vi "main 2.7.22.vi"() -> ()   [LabVIEW 2021]
panel:
  out "Thermistors":cluster{"Filtered x":dbl, "Filtered x":dbl}(graph)
  out "Waveform Chart 3":T1(graph)
  in  "error in (no error)":errorcluster
  out "error out":errorcluster
  out "Waveform Chart 2":waveform(dbl)(graph)
  out "a0 Scalar":dbl
  out "Waveform Chart":dynamicdata(graph)
  in  "stop":bool
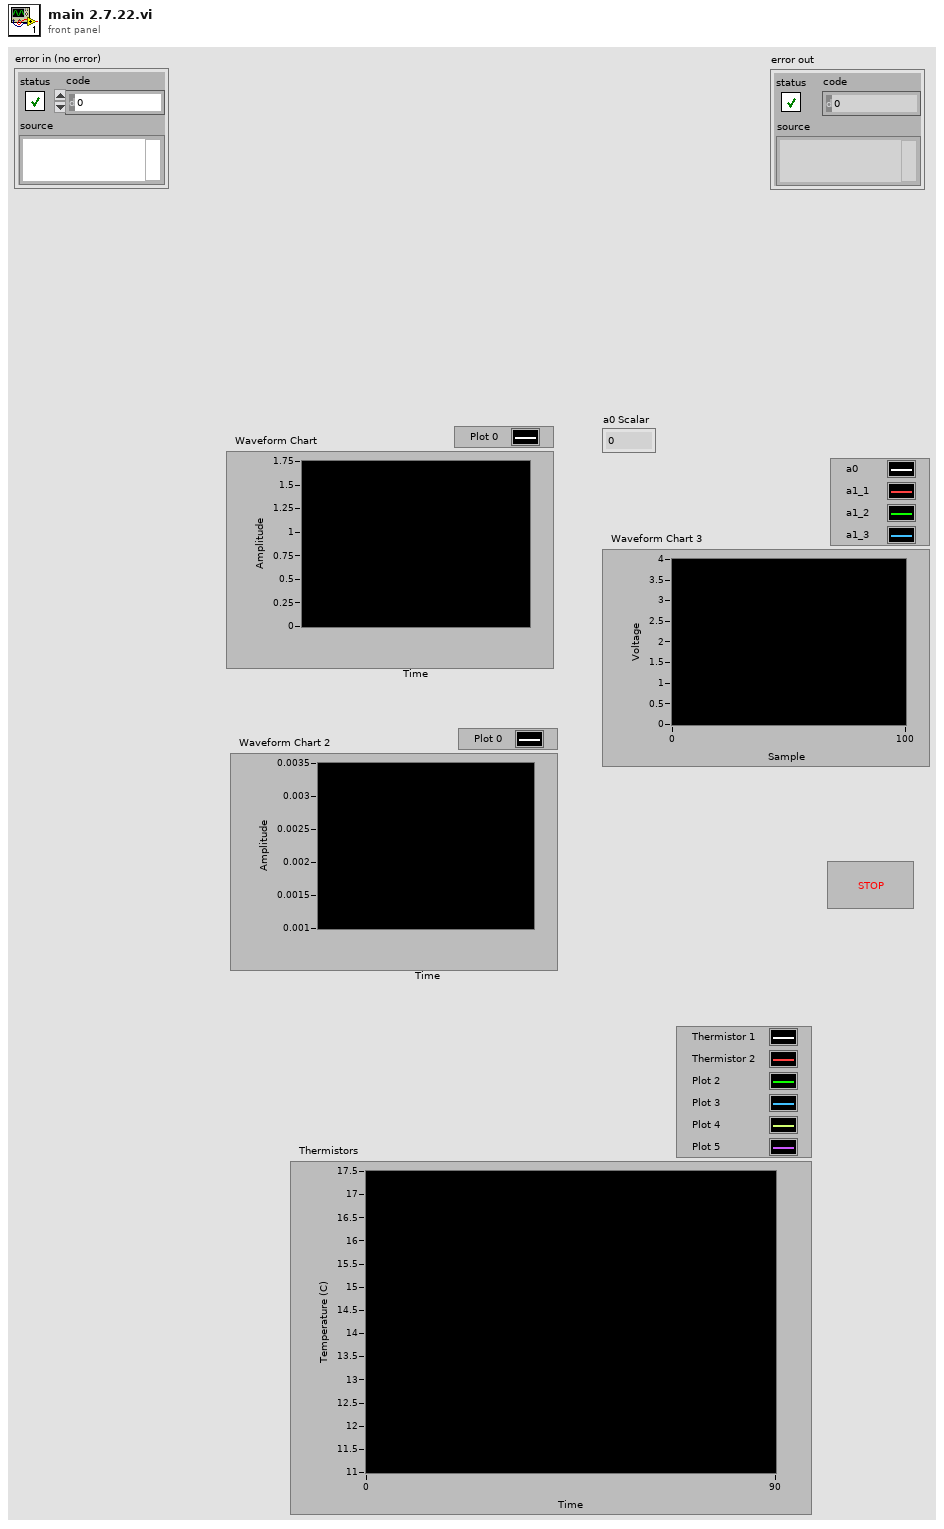
[diagram p1: front panel]
types:
  T1 = cluster{"Data_Array[0]":dbl, "Data_Array[1]":dbl, "Data_Array[2]":dbl, "Data_Array[3]":dbl, "Data_Array[4]":dbl, "Data_Array[5]":dbl, "Data_Array[6]":dbl, "Data_Array[7]":dbl, "Data_Array[8]":dbl}
  T2 = cluster{"Data_Array":dbl[], "Multiplex_Tbl":u32[]}
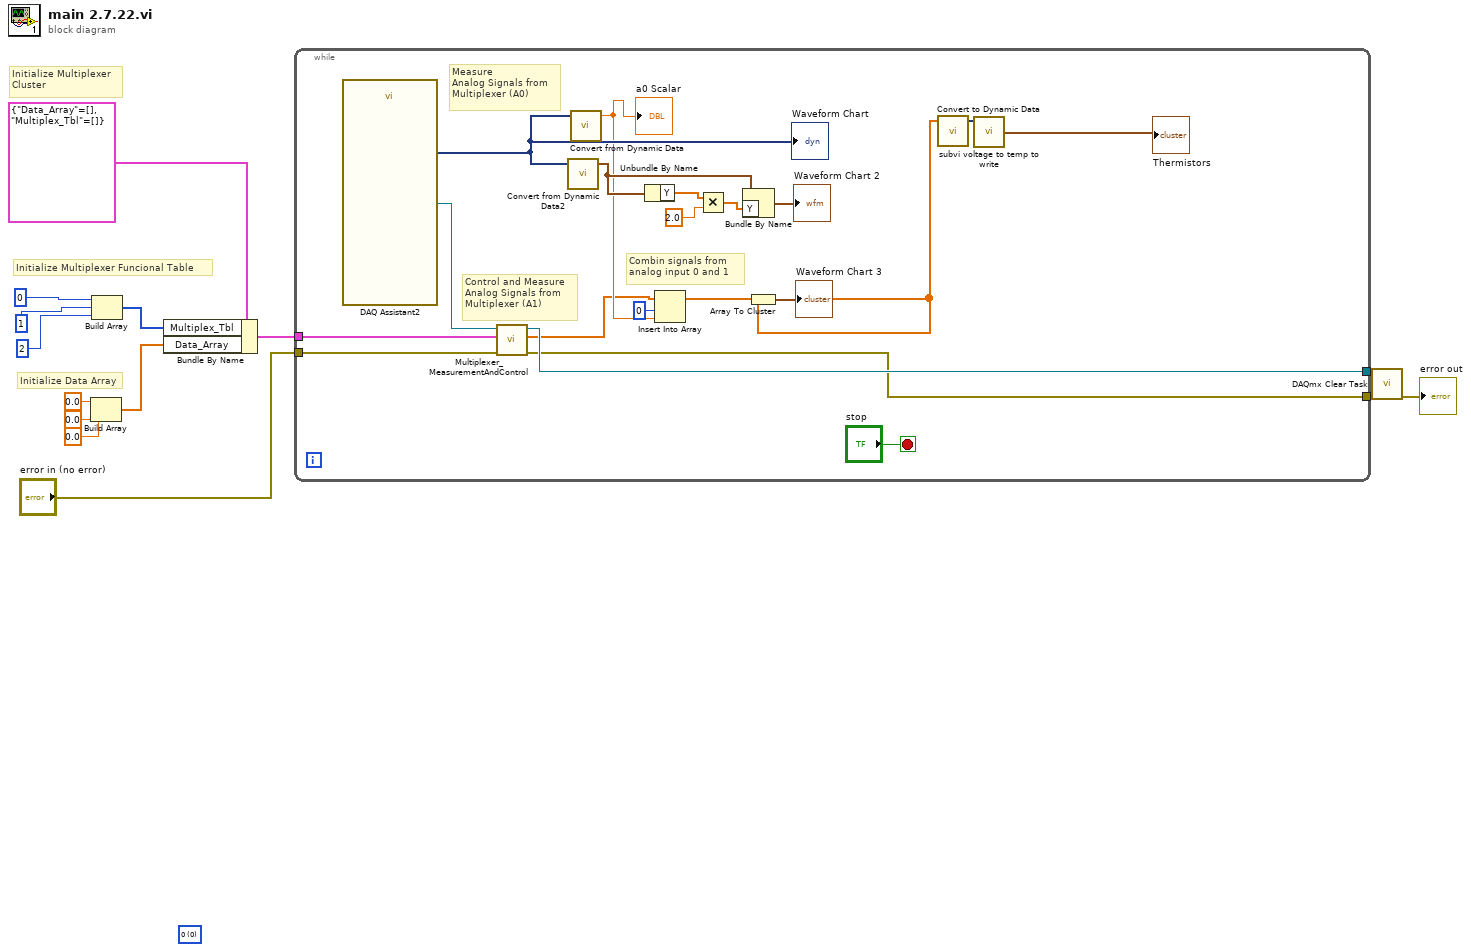
[diagram p0: block diagram]
diagram:
  (unwired) u8 0 items=["0", "1", "Z", "L", "H", "X", "T", "V"] ("digital values ring")
  # "Initialize Multiplexer \nCluster"
  # "Initialize Data Array"
  # "Initialize Multiplexer Funcional Table"
  n1 = Build Array(0.0 ("element"), 0.0 ("element"), 0.0 ("element")) -> (w10:dbl[])
  n2 = Build Array(u32 0 ("Waveform"), 1 ("Waveform"), u32 2 ("Waveform")) -> (w4:u32[])
  n3 = Bundle By Name(cluster=T2 {"Data_Array"=[], "Multiplex_Tbl"=[]}, "Multiplex_Tbl"=w4, "Data_Array"=w10) -> (w9:T2)
  n4 = while {
    tunnel: w9 -> [w26]
    tunnel: "error in (no error)" -> [w25]
    tunnel: [w23] -> w3
    tunnel: [w22] -> w2
    stop <- "stop" stop-if-true
    # "Combin signals from \nanalog input 0 and 1"
    # "Measure\nAnalog Signals from\nMultiplexer (A0)"
    # "Control and Measure\nAnalog Signals from\nMultiplexer (A1)"
    n5 = call "DAQ Assistant2"() -> ("task out"=w24:refnum<k21>, "data"=w27:dynamicdata)  [unwired: 16 in, 2 out]
    "Waveform Chart" <- w27
    n6 = call "Multiplexer_MeasurementAndControl.vi"("error in (no error)"=w25, "Multiplexer_Cluser"=w26, "Task in"=w24) -> ("error out"=w22:errorcluster, "Data_Array"=w19:dbl[], "Task out"=w23:refnum<k21>)  [unwired: 6 in]
    n7 = call "Convert from Dynamic Data2"("Dynamic Data Type"=w27) -> ("Waveform"=w30:waveform(dbl))  [unwired: 3 in]
    n8 = call "Convert from Dynamic Data"("Dynamic Data Type"=w27) -> ("Scalar"=w21:dbl)  [unwired: 3 in]
    "a0 Scalar" <- w21
    n9 = Unbundle By Name(w30) -> ("Y"=w32:dbl[])
    n10 = Insert Into Array(array=w19, index=0, new element=w21) -> (w16:dbl[])
    n11 = Multiply(x=w32, y=2.0) -> (x*y=w29:dbl[])
    n12 = Bundle By Name(cluster=w30, "Y"=w29) -> (→"Waveform Chart 2":waveform(dbl))
    n13 = Array To Cluster(array=w16) -> (cluster=→"Waveform Chart 3":T1)
    n14 = call "Convert to Dynamic Data"("Array"=w16) -> ("Dynamic Data Type"=w15:dynamicdata)  [unwired: 3 in]
    n15 = call "subvi voltage to temp to write.vi"("data"=w15) -> ("Thermistor 1 and 2"=→"Thermistors":cluster{"Filtered x":dbl, "Filtered x":dbl})  [unwired: 10 in]
  }
  n16 = call <vilib>:"DAQmx Clear Task.vi"("task in"=w3, "error in"=w2) -> ("error out"=→"error out":errorcluster)  [unwired: 13 in]
